vi "Close.vi"(8 "error in (no error)":errorcluster, 11 "SLL Database in":refnum<class "SLL Database.lvclass">) -> (0 "error out":errorcluster, 3 "SLL Database out":refnum<class "SLL Database.lvclass">)   [LabVIEW 2016, in "SLL Database.lvclass"]
doc: "Close the Database Connection"
uses:
  SLL Database.lvclass
  SLL Database.lvclass/SLL Database.ctl
  <vilib>/addons/database/NI_Database_API.lvlib
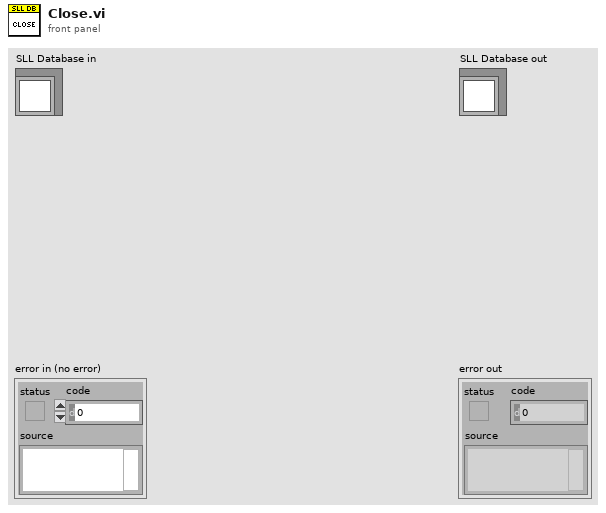
[diagram p1: front panel]
types:
  T1 = typedef "NI_Database_API.lvlib/Conn ObjectReference.ctl" = refnum<k1>
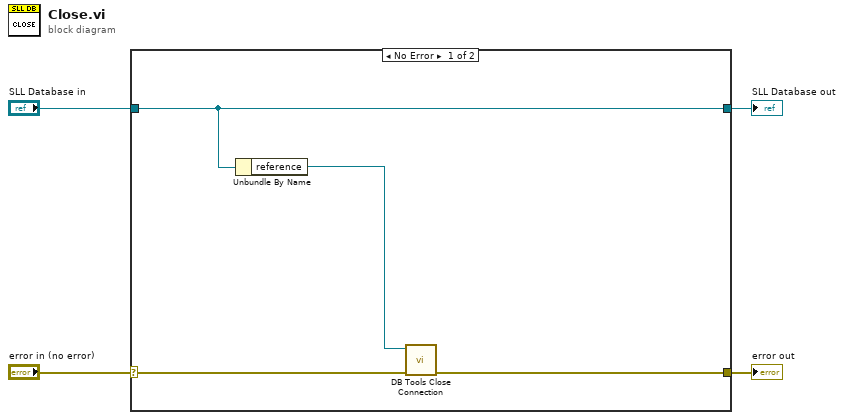
[diagram p0: block diagram]
diagram:
  n1 = case shown="No Error" "error in (no error)" {
    selector: "error in (no error)" -> [w8 w10]
    tunnel: [w7 w10] -> w3
    tunnel: [w6 w9] -> w1
    tunnel: "SLL Database in" -> [w6 w9]
    frame No Error {
      n2 = Unbundle By Name(w6) -> ("reference"=w5:T1)
      n3 = call <vilib>:"DB Tools Close Connection.vi"("error in (no error)"=w8, "connection reference"=w5) -> ("error out"=w7:errorcluster)  [unwired: 5 in]
    }
    frame Error {
    }
  }
  "error out" <- w3
  "SLL Database out" <- w1
